vi "Ejercicio_1_Analizador_Generador_Seno.vi"() -> ()   [LabVIEW 2020]
uses:
  <vilib>/Waveform/WDTOps.llb/WDT Append Waveforms DBL.vi
  <vilib>/measure/maspectr.llb/FFT Power Spectrum and PSD for 1 Chan.vi
  <vilib>/measure/NI_MABase.lvlib
  <vilib>/measure/NI_MAPro.lvlib
panel:
  in  "averaging parameters":T1={"averaging mode"=enum."No averaging", "weighting mode"=enum."Exponential", "number of averages"=10} {"number of averages" min=1}
  in  "sampling info":cluster{"Fs":dbl, "#s":dbl}={"Fs"=1000.0, "#s"=1000.0} {"Fs" format="%.2p"}
  out "Waveform Graph 2":waveform(dbl)(graph)
  out "Waveform Graph":cluster{"f0":dbl, "df":dbl, "magnitude":dbl[]}(graph)
  in  "stop":bool
  in  "Slide 3":dbl(slide) scale=0.0..10.0
  in  "Slide 2":dbl(slide) scale=0.0..10.0
  in  "Slide":dbl(slide) scale=0.0..500.0
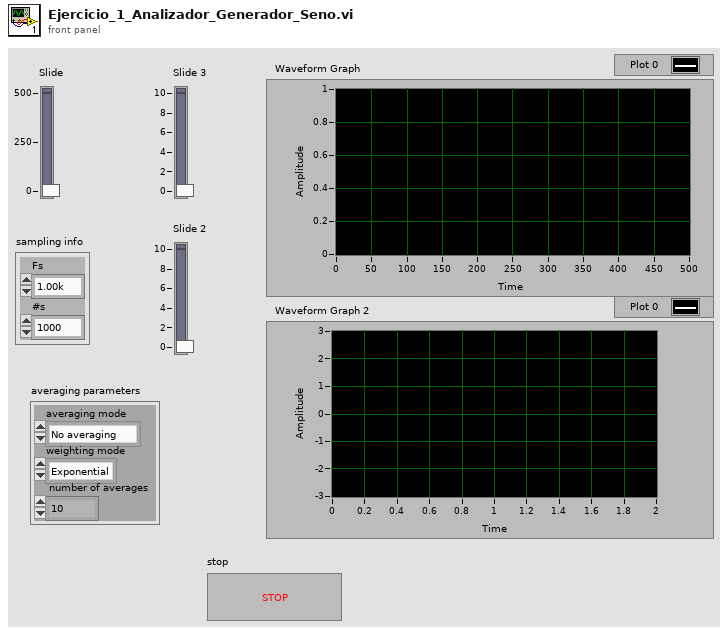
[diagram p1: front panel]
types:
  T1 = cluster{"averaging mode":enum16{"No averaging", "Vector averaging", "RMS averaging", "Peak hold"}, "weighting mode":enum16{"Linear", "Exponential"}, "number of averages":u32}
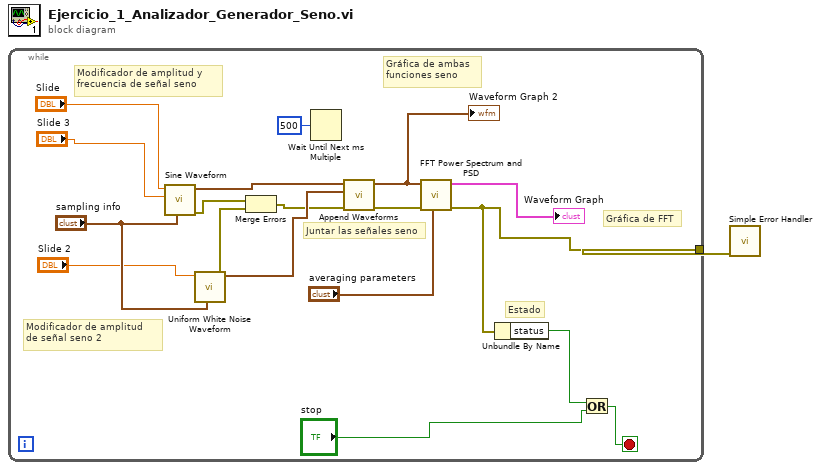
[diagram p0: block diagram]
diagram:
  n1 = while {
    tunnel: [w9] -> w1
    stop <- w6 stop-if-true
    # "Gráfica de FFT"
    # "Gráfica de ambas \nfunciones seno"
    # "Estado"
    # "Juntar las señales seno"
    # "Modificador de amplitud \nde señal seno 2"
    # "Modificador de amplitud y \nfrecuencia de señal seno"
    n2 = call <vilib>:"Sine Waveform.vi"("sampling info"="sampling info", "amplitude"="Slide 3", "frequency"="Slide") -> ("error out"=w17:errorcluster, "signal out"=w14:waveform(dbl))  [unwired: 7 in]
    n3 = call <vilib>:"Uniform White Noise Waveform.vi"("sampling info"="sampling info", "amplitude"="Slide 2") -> ("error out"=w18:errorcluster, "signal out"=w16:waveform(dbl))  [unwired: 8 in]
    n4 = Merge Errors(w17, w18) -> (w15:errorcluster)
    n5 = Wait Until Next ms Multiple(millisecond multiple=u32 500) -> ()  [unwired: 1 out]
    n6 = call-poly <vilib>:"Append Waveforms.vi"("error in (no error)"=w15, "waveform B"=w16, "waveform A"=w14) -> ("error out"=w12:errorcluster, "waveform out"=w10:waveform(dbl))  [unwired: 7 in]
    "Waveform Graph 2" <- w10
    n7 = call-poly <vilib>:"FFT Power Spectrum and PSD.vi"("averaging parameters"="averaging parameters", "error in (no error)"=w12, "time signal"=w10) -> ("error out"=w9:errorcluster, "Power Spectrum / PSD"=→"Waveform Graph":cluster{"f0":dbl, "df":dbl, "magnitude":dbl[]})  [unwired: 5 in, 2 out]
    n8 = Unbundle By Name(w9) -> ("status"=w8:bool)
    n9 = Or(x=w8, y="stop") -> (x .or. y?=w6:bool)
  }
  n10 = call <vilib>:"Simple Error Handler.vi"("error in (no error)"=w1) -> ()  [unwired: 4 in, 5 out]
